vi "issueInfo.get.vi"(11 "ComicVine_class in":refnum<class "series_class.lvclass">) -> (2 "issueInfo":T1[](array[typedef]), 3 "ComicVine_class out":refnum<class "series_class.lvclass">)   [LabVIEW 2024, in "series_class.lvclass"]
uses:
  series_class.lvclass
  comic_class/issueInfo--cluster.ctl
  comic_class/creator--cluster.ctl
  comic_class/character--cluster.ctl
  comic_class/team--cluster.ctl
  comic_class/location--cluster.ctl
  comic_class/concept--cluster.ctl
  comic_class/thing--cluster.ctl
  comic_class/storyArc--cluster.ctl
  series_class.lvclass/series_class.ctl
  issue_class/issue_class.lvclass
  comic_class/comic_class.lvclass
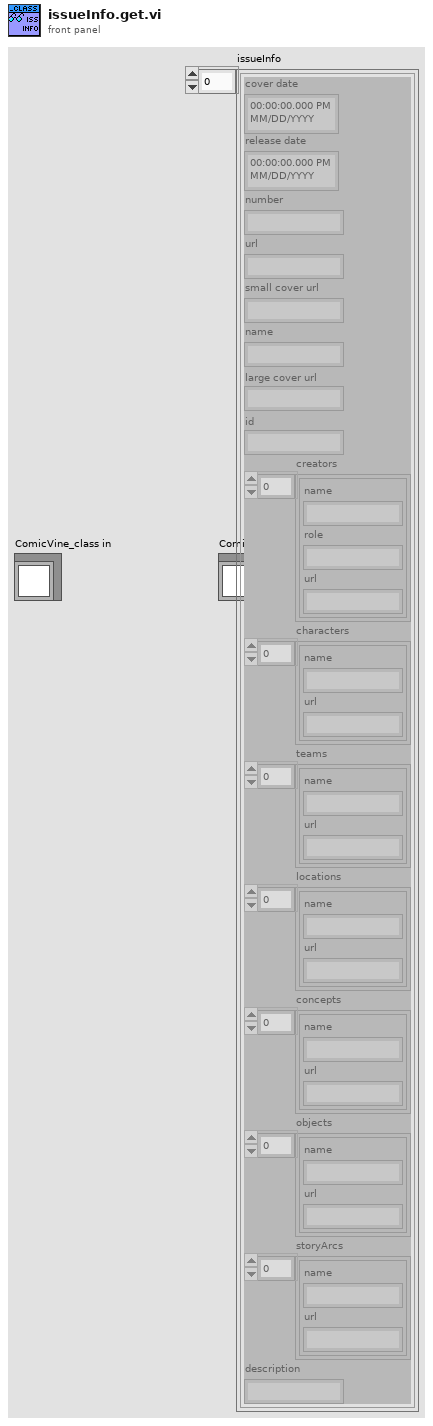
[diagram p1: front panel]
types:
  T1 = typedef "comic_class.lvclass/issueInfo--cluster.ctl" = cluster{"cover date":timestamp, "release date":timestamp, "number":string, "url":string, "small cover url":string, "name":string, "large cover url":string, "id":string, "creators":T2[], "characters":T3[], "teams":T4[], "locations":T5[], "concepts":T6[], "objects":T7[], "storyArcs":T8[], "description":string}
  T2 = typedef "comic_class.lvclass/creator--cluster.ctl" = cluster{"name":string, "role":string, "url":string}
  T3 = typedef "comic_class.lvclass/character--cluster.ctl" = cluster{"name":string, "url":string}
  T4 = typedef "comic_class.lvclass/team--cluster.ctl" = cluster{"name":string, "url":string}
  T5 = typedef "comic_class.lvclass/location--cluster.ctl" = cluster{"name":string, "url":string}
  T6 = typedef "comic_class.lvclass/concept--cluster.ctl" = cluster{"name":string, "url":string}
  T7 = typedef "comic_class.lvclass/thing--cluster.ctl" = cluster{"name":string, "url":string}
  T8 = typedef "comic_class.lvclass/storyArc--cluster.ctl" = cluster{"name":string, "url":string}
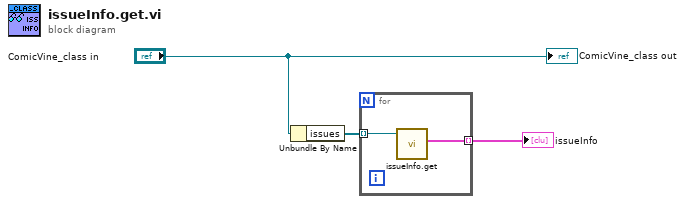
[diagram p0: block diagram]
diagram:
  n1 = Unbundle By Name("ComicVine_class in") -> ("issues"=w2:refnum<class "issue_class.lvclass">[])
  n2 = for {
    tunnel: w2 -> [w5] mode=indexing
    tunnel: [w4] -> w1 mode=indexing
    n3 = call "issueInfo.get.vi"("issue_class in"=w5) -> ("issueInfo"=w4:T1)  [unwired: 9 in, 1 out]
  }
  "issueInfo" <- w1
  "ComicVine_class out" <- "ComicVine_class in"
